vi "Assignment3_ProductSpecifications.vi"() -> ()   [LabVIEW 2024]
panel:
  in  "stop":bool
  out "Product Specifications":T1
  in  "Make":enum16{"Samsung", "LG", "Bosch"}(ring)
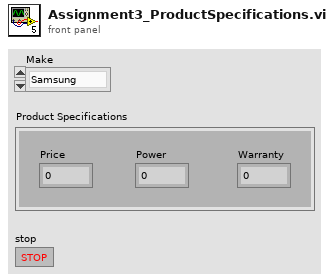
[diagram p1: front panel]
types:
  T1 = cluster{"Price":dbl, "Power":dbl, "Warranty":dbl}
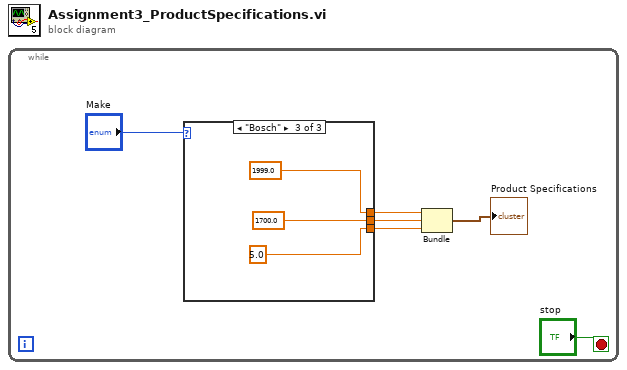
[diagram p0: block diagram]
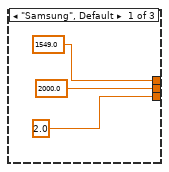
[diagram p2: hidden frame]
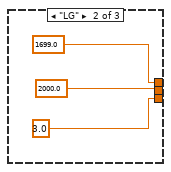
[diagram p3: hidden frame]
diagram:
  n1 = while {
    stop <- "stop" stop-if-true
    n2 = case shown="\"Bosch\"" "Make" {
      tunnel: [1549.0 1699.0 1999.0] -> w4
      tunnel: [2000.0 2000.0 1700.0] -> w3
      tunnel: [2.0 3.0 5.0] -> w2
      frame "Samsung", Default {
      }
      frame "LG" {
      }
      frame "Bosch" {
      }
    }
    n3 = Bundle(w4, w3, w2) -> (→"Product Specifications":cluster{dbl, dbl, dbl})  [unwired: 1 in]
  }
